vi "SS_ErrorHandler.vi"(6 "Main Cluster IN":T1, 8 "Error In":errorcluster, 9 "SubVI Error":errorcluster, 10 "SubVI Name":string, 11 "Info In":string="\nWaiting for TimerScope Trigger\n- IN: SS TimerScope Trigger\n- OUT: SET SS ThermoRec Received Trigger\nPulse Number is 231123\nPulse Type is 4\n\nDuration (s) is  2.000000\nDelay (s)  is  1.000000\nScan Period (ms) is  15\nNumber of Samples is  134\n\nDelay Started\nDelay Complete\nExternal Measurement of Delay (s): 1.000000\nACQUIRING DATA") -> (0 "Error Out":errorcluster, 3 "Info Out":string="\nWaiting for TimerScope Trigger\n- IN: SS TimerScope Trigger\n- OUT: SET SS ThermoRec Received Trigger\nPulse Number is 231123\nPulse Type is 4\n\nDuration (s) is  2.000000\nDelay (s)  is  1.000000\nScan Period (ms) is  15\nNumber of Samples is  134\n\nDelay Started\nDelay Complete\nExternal Measurement of Delay (s): 1.000000\nACQUIRING DATA", 4 "Main Cluster OUT":T1)   [LabVIEW 2016]
uses:
  Control/Control_Main.ctl
  Control/Control_ModuleArray.ctl
panel:
  in  "Tab Control":enum32{"IN", "OUT", "SubVI Info"}(tab)
  out "Error String In":string
  out "Error String Out":string
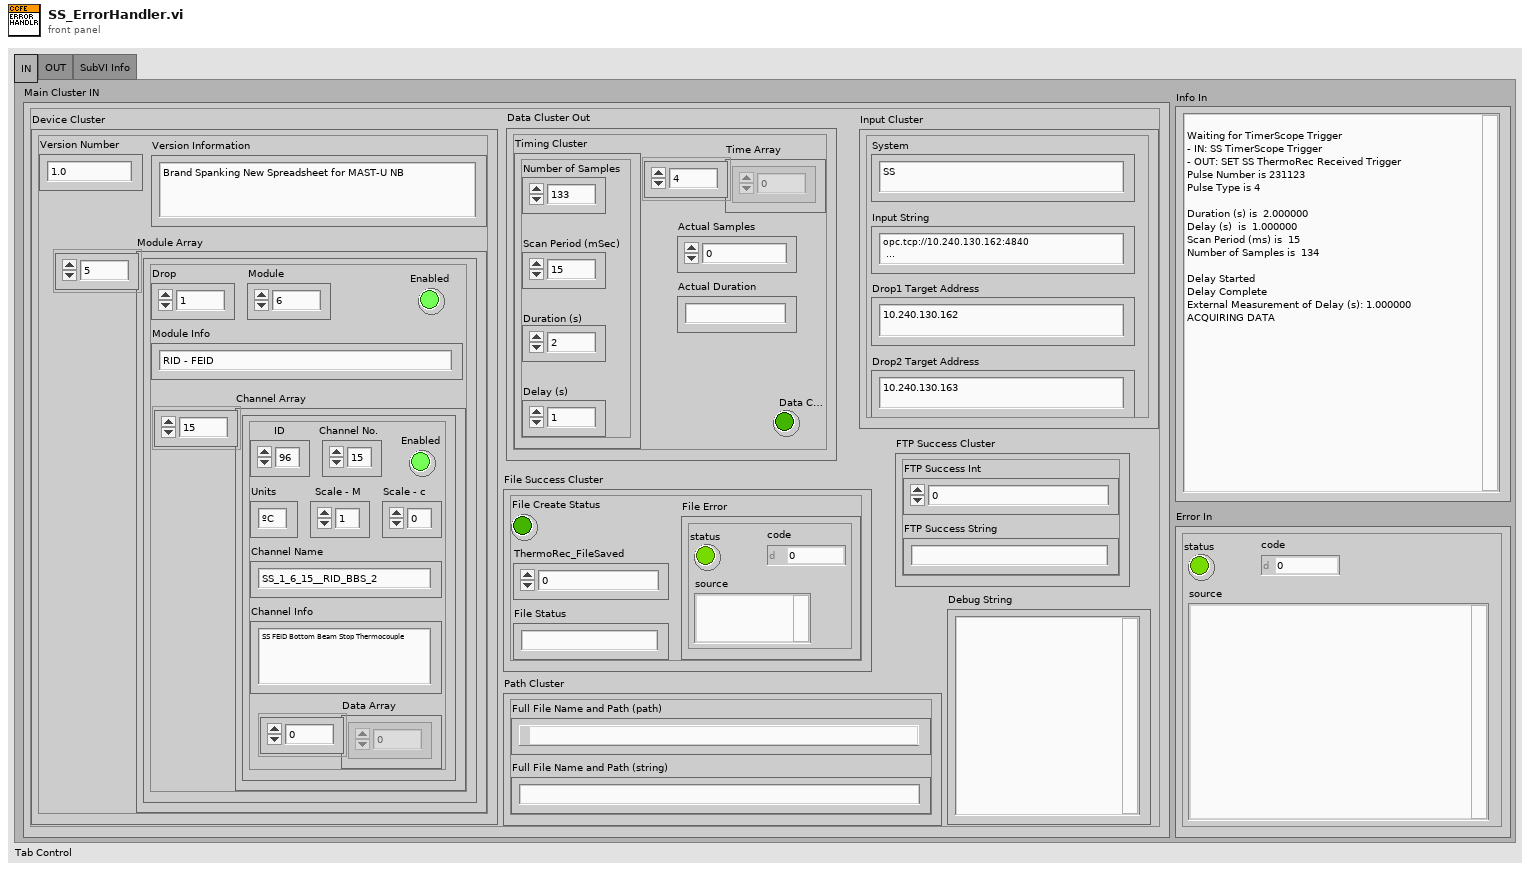
[diagram p1: front panel]
types:
  T1 = typedef "Control_Main.ctl" = cluster{"Device Cluster":cluster{"Module Array":T2, "Version Number":string, "Version Information":string}, "Input Cluster":cluster{"Input String":string, "Drop1 Target Address":string, "Drop2 Target Address":string, "System":string}, "Data Cluster Out":cluster{"Timing Cluster":cluster{"Number of Samples":i32, "Scan Period (mSec)":u32, "Duration (s)":dbl, "Delay (s)":dbl}, "Time Array":dbl[], "Actual Samples":i32, "Actual Duration":string, "Data Collection Error":bool}, "Path Cluster":cluster{"Full File Name and Path (path)":path, "Full File Name and Path (string)":string}, "File Success Cluster":cluster{"ThermoRec_FileSaved":i32, "File Create Status":bool, "File Error":errorcluster, "File Status":string}, "FTP Success Cluster":cluster{"FTP Success Int":i32, "FTP Success String":string}, "Debug String":string}
  T2 = typedef "Control_ModuleArray.ctl" = cluster{"Drop":i32, "Module":i32, "Module Info":string, "Enabled":bool, "Channel Array":cluster{"ID":i32, "Channel No.":i32, "Enabled":bool, "Channel Name":string, "Channel Info":string, "Units":string, "Scale - M":dbl, "Scale - c":dbl, "Data Array":dbl[]}[]}[]
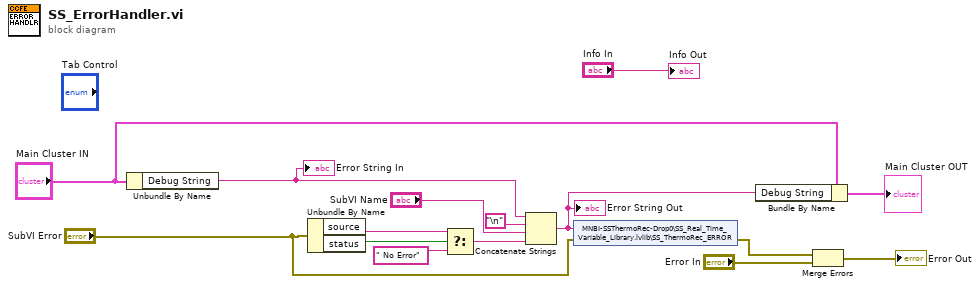
[diagram p0: block diagram]
diagram:
  n1 = Unbundle By Name("Main Cluster IN") -> ("Debug String"=w8:string)
  "Error String In" <- w8
  n2 = Unbundle By Name("SubVI Error") -> ("source"=w10:string, "status"=w12:bool)
  n3 = Select(t=w10, s=w12, f=" No Error") -> (s? t:f=w11:string)
  n4 = Concatenate Strings(w8, "\n", "SubVI Name", w11) -> (w2:string)
  "Error String Out" <- w2
  n5 = shared-variable "MNBI-SSThermoRec-Drop0\\SS_Real_Time_Variable_Library.lvlib\\SS_ThermoRec_ERROR"(w2, error in="SubVI Error") -> (error out=w14:errorcluster)
  n6 = Bundle By Name(cluster="Main Cluster IN", "Debug String"=w2) -> (→"Main Cluster OUT":T1)
  n7 = Merge Errors(w14, "Error In") -> (→"Error Out":errorcluster)
  "Info Out" <- "Info In"
